vi "PicoScope5000aExampleStreaming.vi"() -> ()   [LabVIEW 2015]
uses:
  ps5000a.dll
panel:
  out "Triggered":bool
  out "Sample Interval":u32
  in  "Acquisition Settings":T1={"Auto Stop"=TRUE, "Four Channel Device?"=FALSE, "Desired Sample Interval"=1, "Pre-trigger Samples"=0, "Post-trigger Samples"=1000000, "Down-Sample Ratio"=1, "Down-Sample Mode"=0, "Overview Buffer Size"=100000, "Time Units"=3} {"Time Units" items=["Nanoseconds (ns)"=2, "Microseconds (us)"=3, "Milliseconds (ms)"=4, "Seconds (s)"=5]; "Down-Sample Mode" items=["None"=0, "Aggregate"=1, "Decimate"=2, "Average"=4]}
  out "Total Samples":u32
  out "Auto Stopped":bool
  in  "Serial Number":string
  in  "Open Using Serial Number":bool
  out "Number of Samples per Capture":u32
  in  "Resolution":i32(ring) items=["8-bit", "12-bit", "14-bit", "15-bit (max. 2 ch.)", "16-bit (max. 1 ch.)"]
  in  "Trigger Settings":T2={"Trigger Enabled"=TRUE, "Trigger Source"=enum."Channel A", "Trigger Threshold (16-bit counts)"=16384, "Trigger Direction"=2, "Trigger Delay (samples)"=0, "Auto Trigger Time (ms)"=0} {"Trigger Direction" items=["Rising"=2, "Falling"=3]}
  in  "PS5X4XA/B devices\nUSB Powered":bool=TRUE
  in  "Channel A Settings":T3={"Enabled"=TRUE, "Coupling"=1, "Range"=7, "Analogue Offset"=0.0} {"Range" items=["10 mV", "20 mV", "50 mV", "100 mV", "200 mV", "500 mV", "1 V", "2 V", "5 V", "10 V", "20 V", "50 V ", "100 V"]; "Coupling" items=["AC", "DC"]}
  in  "Apply  Settings":bool
  out "Channel A":i16[](graph)
  in  "stop":bool
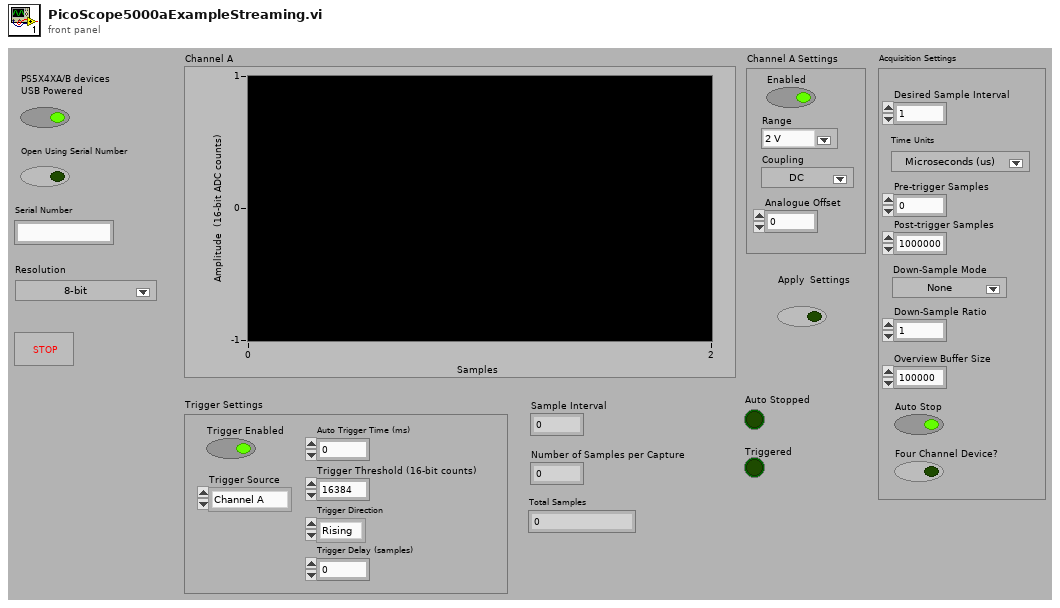
[diagram p1: front panel]
types:
  T1 = cluster{"Auto Stop":bool, "Four Channel Device?":bool, "Desired Sample Interval":u32, "Pre-trigger Samples":u32, "Post-trigger Samples":u32, "Down-Sample Ratio":u32, "Down-Sample Mode":i32, "Overview Buffer Size":u32, "Time Units":u32}
  T2 = cluster{"Trigger Enabled":bool, "Trigger Source":enum16{"Channel A", "Channel B", "Channel C", "Channel D", "Ext."}, "Trigger Threshold (16-bit counts)":i16, "Trigger Direction":u16, "Trigger Delay (samples)":u32, "Auto Trigger Time (ms)":i16}
  T3 = cluster{"Enabled":bool, "Coupling":i16, "Range":u16, "Analogue Offset":sgl}
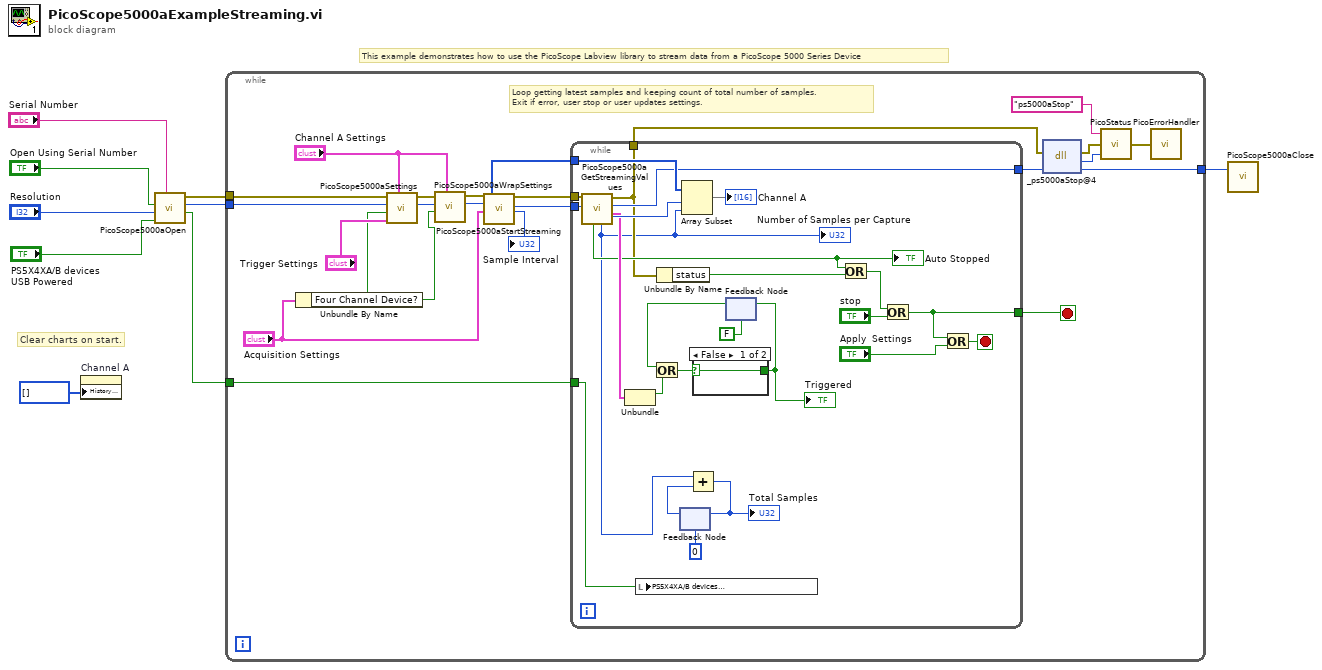
[diagram p0: block diagram]
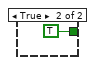
[diagram p2: hidden frame]
diagram:
  # "Clear charts on start."
  # "This example demonstrates how to use the PicoScope Labview library to stream data from a PicoScope 5000 Series Device"
  n1 = property on="Channel A" class="WFChart (strict)"("History Data"=i16[] []) -> ()  [unwired: 2 in, 2 out]
  n2 = call "PicoScope5000aOpen.vi"("Serial Number"="Serial Number", "USB Powered Selection"="PS5X4XA/B devices\nUSB Powered", "Resolution"="Resolution", "Use Serial Number"="Open Using Serial Number") -> ("USB Powered Indication"=w3:bool, "handle"=w8:i16, "error out"=w9:errorcluster)  [unwired: 2 in, 1 out]
  n3 = while {
    tunnel: [w24] -> w1
    tunnel: w9 -> [w30]
    tunnel: w8 -> [w31]
    tunnel: w3 -> [w18]
    stop <- w32 stop-if-true
    # "Loop getting latest samples and keeping count of total number of samples. \nExit if error, user stop or user updates settings."
    n4 = Unbundle By Name("Acquisition Settings") -> ("Four Channel Device?"=w13:bool)
    n5 = call "PicoScope5000aSettings.vi"("Channel A Settings"="Channel A Settings", "Trigger Settings"="Trigger Settings", "Four Channel Device?"=w13, "handle in"=w31, "error in"=w30) -> ("handle out"=w14:i16, "error out"=w15:errorcluster)  [unwired: 5 in]
    n6 = call "PicoScope5000aWrapSettings.vi"("Channel A Settings"="Channel A Settings", "Four Channel Device?"=w13, "Handle In"=w14, "error in (no error)"=w15) -> ("Handle Out"=w17:i16, "error out"=w16:errorcluster)  [unwired: 6 in]
    n7 = call "PicoScope5000aStartStreaming.vi"("error in"=w16, "handle in"=w17, "Acquisition Settings"="Acquisition Settings") -> ("Channel A"=w29:i16[], "error out"=w27:errorcluster, "handle out"=w28:i16, "Sample Interval"=→"Sample Interval":u32)  [unwired: 6 in, 7 out]
    n8 = while {
      tunnel: [w51] -> w25
      tunnel: [w55] -> w32
      tunnel: w29 -> [w53]
      tunnel: w28 -> [w49]
      tunnel: w27 -> [w48]
      tunnel: w18 -> [w47]
      tunnel: [w42] -> w23
      stop <- w54 stop-if-true
      n9 = call "PicoScope5000aGetStreamingValues.vi"("handle in"=w49, "error in"=w48) -> ("Start Index in Driver Buffer"=w50:u32, "Trigger"=w46:cluster{bool, "triggeredAt (Total samples)":u32}, "handle out"=w51:i16, "error out"=w42:errorcluster, "Number of Samples"=w34:u32, "Auto Stopped"=w43:bool)  [unwired: 4 in]
      "Number of Samples per Capture" <- w34
      "Auto Stopped" <- w43
      n10 = Unbundle(w46) -> (w35:bool)  [unwired: 1 out]
      n11 = local write "PS5X4XA/B devices\nUSB Powered"(w47) -> ()
      n12 = Unbundle By Name(w42) -> ("status"=w45:bool)
      n13 = feedback #1(u32 0) -> (w33:u32)
      n14 = Array Subset(array=w53, index=w50, length=w34) -> (→"Channel A":i16[])
      n15 = Add(x=w34, y=w33) -> (x+y=w40:u32)
      "Total Samples" <- w40
      n16 = feedback-in #1(w40) -> ()
      n17 = feedback #2(FALSE) -> (w38:bool)
      n18 = Or(x=w38, y=w35) -> (x .or. y?=w37:bool)
      n19 = case shown="False" w37 {
        selector: w37 -> [w58 _]
        tunnel: [w58 TRUE] -> w39
        frame False {
        }
        frame True {
        }
      }
      "Triggered" <- w39
      n20 = feedback-in #2(w39) -> ()
      n21 = Or(x=w43, y=w45) -> (x .or. y?=w44:bool)
      n22 = Or(x=w44, y="stop") -> (x .or. y?=w55:bool)
      n23 = Or(x=w55, y="Apply  Settings") -> (x .or. y?=w54:bool)
    }
    n24 = dll-call lib="C:/Labview/2015.10.08_Rydberg_ExpControl/PicoScope/LV_Driver/ps5000a.dll" fn="_ps5000aStop@4"(error in=w23, "handle"=w25) -> (error out=w21:errorcluster, "PICO_STATUS"=w22:u32, "handle"=w24:i16)  [unwired: 2 in, 1 out]
    n25 = call "PicoStatus.vi"("PICO STATUS"=w22, "error in"=w21, "source"="ps5000aStop") -> ("error out"=w20:errorcluster)
    n26 = call "PicoErrorHandler.vi"("error in"=w20) -> ()  [unwired: 1 out]
  }
  n27 = call "PicoScope5000aClose.vi"("handle"=w1) -> ()  [unwired: 2 in, 1 out]
